vi "Treat DIGITAL variables.vi"(0 "Analog Variable info fixed":T3[](array[typedef]), 1 "Common alarm handling(F)":bool, 5 "All issues in Alm list":bool, 7 "Status Values":T13[](array[typedef]), 9 "Variabel start index":i32, 11 "error In":errorcluster, 12 "Analog Variable info Settings":T6[](array[typedef])) -> (3 "Categorized  Status":T1[](array[typedef]), 4 "Digital Variable Display":T10[](array[typedef]), 6 "Action":T8, 8 "Digital status Values":T13[](array[typedef]), 10 "Alarms":bool[](array[boolean]), 14 "Issue Alarm strings":string[][](array[string]), 15 "error out":errorcluster)   [LabVIEW 2011]
uses:
  Action List.ctl
  Status Digitalish.ctl
  Digital GUI/Digital Display cluster.ctl
  Digital GUI/Digital Disp small indicator.ctl
  GUI/Status indicator white.ctl
  User Setting DigitalChannel.ctl
  Alarm Responce.ctl
  Alarm Responce dig.ctl
  Fixed Digital Channel Definition.ctl
  Update frequensies.ctl
  Channel catagory Enum.ctl
  Catagorised alarm state.ctl
  GUI/Status Indikator Helper.ctl
  Application Structure/Options/Action GFV Settings.ctl
  emi cndiates/E&S/reate/S&E Digital Alarm Type.ctl
  emi Lib/System 01/0 - General/emi_Read System ID.vi
  <vilib>/Utility/VariantDataType/GetNumericInfo.vi
  emi Lib/System 01/0 - General/Private/_emi_GFV System ID.vi
  emi Lib/System 01/0 - General/S&E reporting/Private/_emi_S&E Q Generator.vi
  <vilib>/Utility/error.llb/Clear Errors.vi
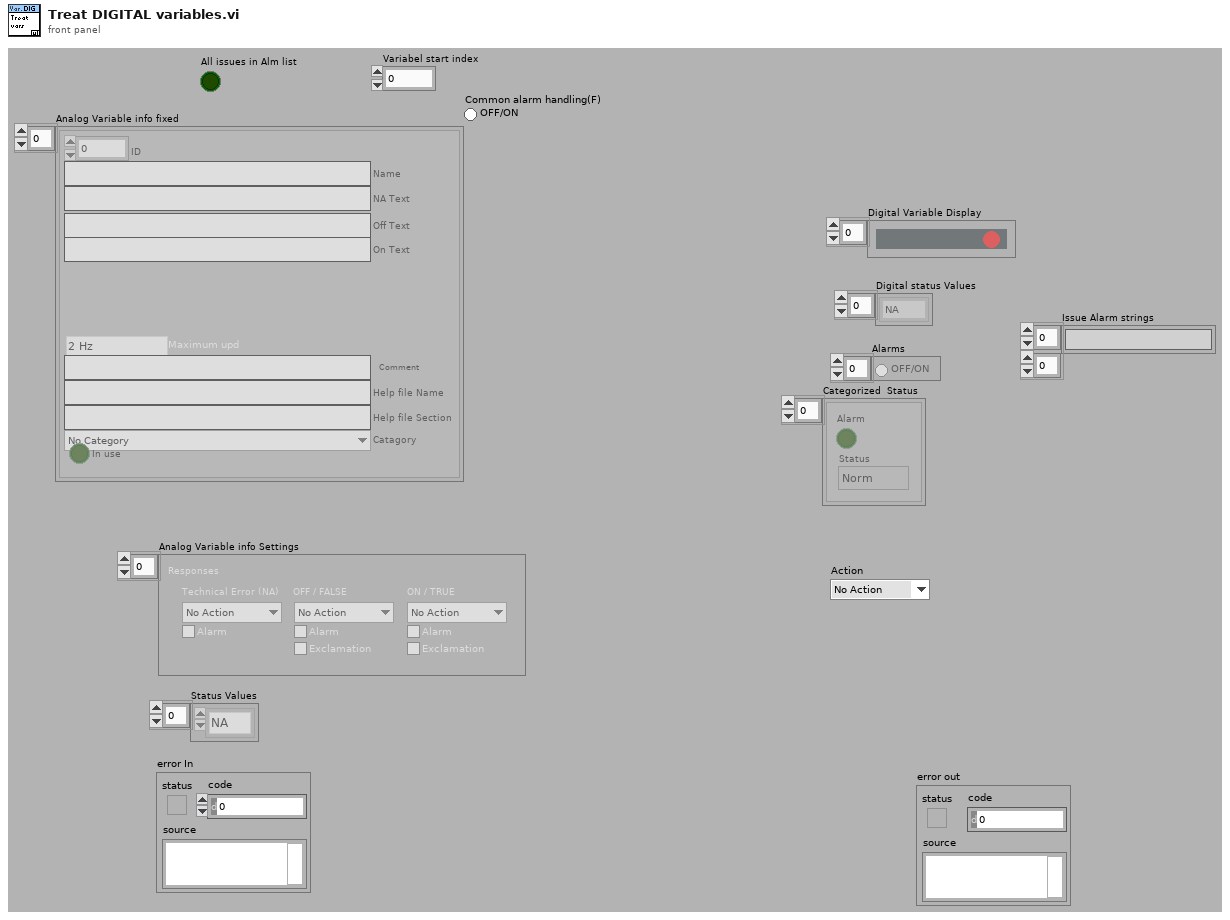
[diagram p1: front panel]
types:
  T1 = typedef "Catagorised alarm state.ctl" = cluster{"Alarm":bool, "Status":T2}
  T2 = typedef "Status Indikator Helper.ctl" = enum16{"Norm", "L", "H", "LL", "HH", "Value", "Technical"}
  T3 = typedef "Fixed Digital Channel Definition.ctl" = cluster{"ID":u16, "Name":string, "NA Text":string, "Off Text":string, "On Text":string, "Maximum upd":T4, "Comment":string, "Help file Name":string, "Help file Section ":string, "Catagory":T5, "In use":bool}
  T4 = typedef "Update frequensies.ctl" = enum16{"2 Hz", "1 Hz", "0.1 Hz"}
  T5 = typedef "Channel catagory Enum.ctl" = enum16{"No Category", "Power", "Temperature", "Pressure"}
  T6 = typedef "User Setting DigitalChannel.ctl" = cluster{"Responses":cluster{"Technical Error (NA)":T7, "OFF / FALSE":T9, "ON / TRUE":T9}}
  T7 = typedef "Alarm Responce.ctl" = cluster{"Action":T8, "Alarm":bool}
  T8 = typedef "Action List.ctl" = enum16{"No Action", "Stop Motor", "Turn Off HV"}
  T9 = typedef "Alarm Responce dig.ctl" = cluster{"Action":T8, "Alarm":bool, "Exclamation":bool}
  T10 = typedef "Digital Display cluster.ctl" = cluster{"ON/OFF TEXT":string, "Val":T11, "Status":T12}
  T11 = typedef "Digital Disp small indicator.ctl" = u16
  T12 = typedef "Status indicator white.ctl" = u16
  T13 = typedef "Status Digitalish.ctl" = enum16{"NA", "False", "True"}
  T14 = typedef "Action GFV Settings.ctl" = enum16{"Init", "Get From INI", "Put In INI", "Get Settings", "Get Update Index", "Set Setting"}
  T15 = typedef "Options  All pages and custom.ctl" = cluster{"P 1 (App)":T16, "P 2":T17, "P 3":T18, "P 4":T21, "P 5":T26, "P 6 (Err)":T27, "P 7 (Expert)":T28, "P 8 (Depth)":T30, "C 1":T31, "C 2":T32}
  T16 = typedef "Options Page 1 (App).ctl" = cluster{"Result files":path, "PCP Interface":string, "Tractor/Stroker Interface":string, "Tractor Interface":string, "Modem Status Interface":string, "Audible Alarm":bool, "Force alarm on Technical":bool, "Force alarm on HH":bool, "Force alarm on LL":bool, "Force alarm on H":bool, "Force alarm on L":bool}
  T17 = typedef "Options Page 2.ctl" = cluster{"Solenoid & Relay latching time":u16, "Tractor relay 1":dbl, "Tractor relay 2":dbl, "Tractor Solenoid limit":dbl}
  T18 = typedef "Options Page 3.ctl" = cluster{"Min resistance":dbl, "Max resistance":dbl, "Head voltage range":T19, "Max voltage jump":dbl, "Maximum resistance change":dbl, "Start Telemetry Voltage":dbl, "Start Telemetry Timeout":dbl, "Start Motor Voltage":dbl, "Stop Motor Voltage":dbl, "Pass Mode Warning Voltage":dbl, "Relay Switch Voltage":dbl, "Relay Status Loss Voltage":dbl, "Samples to average":i32, "PSU type DO NOT USE":T20, "Magna OVP":dbl, "Magna Current Limit":dbl}
  T19 = typedef "PCP type List.ctl" = enum16{"0 - 350V", "0 - 450V", "0 - 600V"}
  T20 = typedef "PSU Type.ctl" = enum16{"Unipower", "Magna 8.3A", "Magna 12A", "None"}
  T21 = typedef "Options Page 4.ctl" = cluster{"Solenoid & Relay latching time":u16, "Stroker relay 1":dbl, "Stroker Relay 2":dbl, "Stroker Solenoid limit":dbl, "Force det.":T22, "Stroke force lim.":dbl, "Anchor Enabled Pressure":dbl, "Tacometer puls":dbl, "Default anchor behavior":T23, "Default stroker behavior":T24, "Default stroker force limit (tonne)":dbl, "Slips Size":T25}
  T22 = typedef "Stroke force selector.ctl" = enum16{"Stroke in = node 1", "Strok out = node 1"}
  T23 = typedef "Default anchor behavior.ctl" = enum16{"Do nothing", "Set Anchor", "Release Anchor"}
  T24 = typedef "Default stroker behavior.ctl" = enum16{"Do nothing", "Stop", "Go Out", "Go In"}
  T25 = typedef "Slips Type Radio.ctl" = enum32{"No Selection", "338 MRS", "3,9 MRS"}
  T26 = typedef "Options Page 5.ctl" = cluster{"Solenoid & Relay latching time":u16, "Driller relay 1":dbl, "Driller Relay 2":dbl, "Driller  Solenoid limit":dbl}
  T27 = typedef "Options Page 6 (Err).ctl" = cluster{"Error and event files":path}
  T28 = typedef "Options Page 7 (Expert).ctl" = cluster{"Show Debug":bool, "Log debug messages":bool, "Additional debug messages":bool, "Start Beagle with Simulator data":bool, "Workshop mode":bool, "Modem baud":u16, "enumCANCOM":bool, "Modem sim":T29, "Telemetry Timeout Disable":i32, "Buffer size":i32, "Upd regular data":bool, "Cable comp":cluster{"VMOD1 Voltage(V)":dbl, "VMOD2 Voltage(V)":dbl}}
  T29 = typedef "Modem simulation setup.ctl" = cluster{"Modem dealay sim":bool, "Sim baud Tx":u16, "Bit Error fraction Tx":dbl, "Sim baud Rx":u16, "Bit Error fraction Rx":dbl}
  T30 = typedef "Options Page 8 (Depth).ctl" = cluster{"Winch Spool Circumference":dbl, "Winch Pulses per Revolution":dbl, "Current Depth":dbl}
  T31 = typedef "Options Custom 1.ctl" = cluster{"Depth Updated":bool, "Depth Offset":dbl}
  T32 = typedef "Options Custom 2.ctl" = cluster{"Placeholder":bool}
  T33 = typedef "S&E Digital Alarm Type.ctl" = cluster{"Alarm":bool, "Enum":T2, "Value":T13, "Source name":string, "Status text":string}
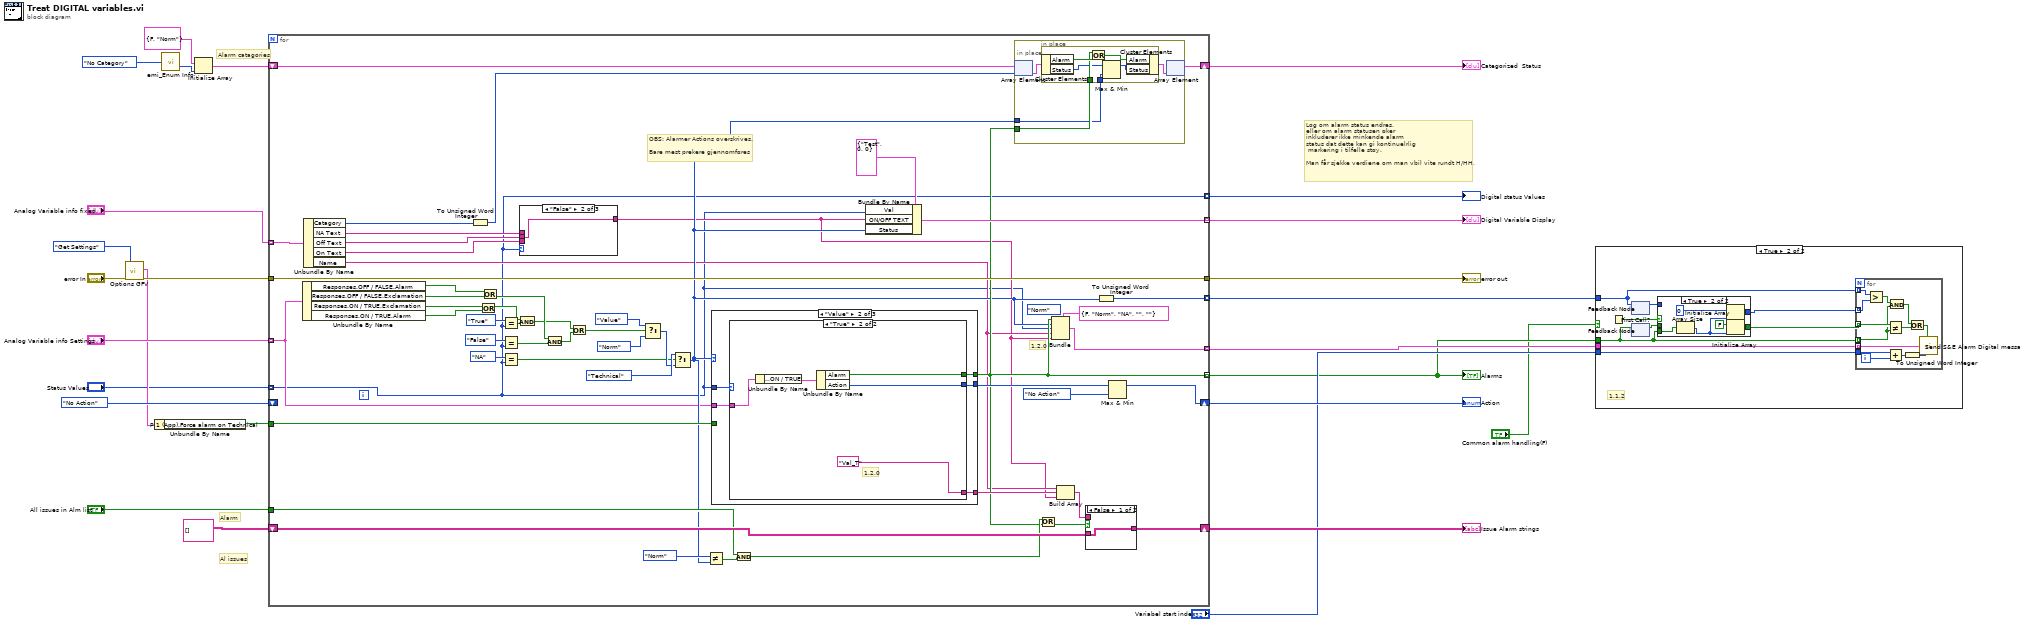
[diagram p0: block diagram]
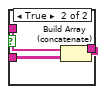
[diagram p6: hidden frame]
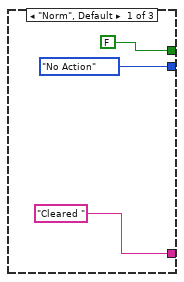
[diagram p7: hidden frame]
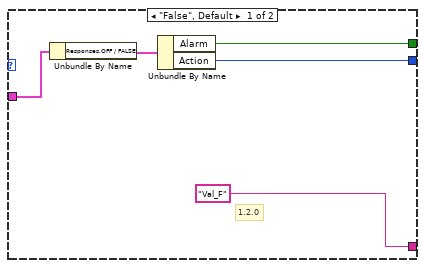
[diagram p8: hidden frame]
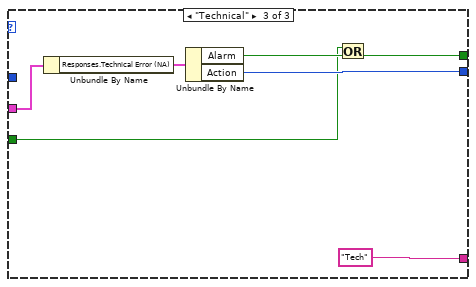
[diagram p9: hidden frame]
diagram:
  # "Log om alarm status endres, \neller om alarm statusen øker\ninkluderer ikke minkende alarm \nstatus dat dette kan gi kontinuelrlig\n markering i tilfelle støy.\n\nMan får sjekke verdiene om man vbil vite rundt H/HH,"
  # "Al issues"
  # "Alarm"
  # "Alarm catagories"
  n1 = call "Options GFV.vi"("error in (no error)"="error In", "Action(Get Settings)"=Action_GFV_Settings."Get Settings") -> ("Options"=w16:T15, "error out"=w18:errorcluster)  [unwired: 15 in, 1 out]
  n2 = Unbundle By Name(w16) -> ("P 1 (App).Force alarm on Technical"=w15:bool)
  n3 = call "emi_Enum Info.vi"("Enum"=Channel_catagory_Enum."No Category" ("Catagory")) -> ("Numb Elements"=w8:i32)  [unwired: 11 in, 3 out]
  n4 = Initialize Array(T1 {"Alarm"=FALSE, "Status"=enum."Norm"} ("catagori"), w8) -> (w6:T1[])
  n5 = for {
    tunnel: "Analog Variable info Settings" -> [w50] mode=indexing
    tunnel: "Analog Variable info fixed" -> [w78] mode=indexing
    tunnel: w18 -> [w74]
    tunnel: [w59] -> w3 mode=indexing
    tunnel: [w75] -> w23 mode=indexing
    tunnel: [w74] -> w24
    shift-right: [w71] -> w26
    shift-left: Action_List."No Action" ("Action") -> [_]
    tunnel: w15 -> [w70]
    shift-right: [w68] -> w14
    shift-left: string[][] [] -> [w67]
    tunnel: "All issues in Alm list" -> [w62]
    tunnel: [w58] -> w11 mode=indexing
    tunnel: [w56] -> w9 mode=indexing
    shift-right: [w54] -> w5
    shift-left: w6 -> [w55]
    tunnel: [w27] -> w4 mode=indexing
    tunnel: "Status Values" -> [w27] mode=indexing
    (unwired) Status_Indikator_Helper."Norm" ("s? t:f")
    # "1.2.0"
    # "OBS: Alarmer Actions overskrives.\n\nBare mest prekere gjennomføres"
    n6 = Unbundle By Name(w50) -> ("Responses.OFF / FALSE.Alarm"=w40:bool, "Responses.OFF / FALSE.Exclamation"=w45:bool, "Responses.ON / TRUE.Exclamation"=w42:bool, "Responses.ON / TRUE.Alarm"=w38:bool)
    n7 = Unbundle By Name(w78) -> ("Catagory"=w33:T5, "NA Text"=w32:string, "Off Text"=w31:string, "On Text"=w30:string, "Name"=w29:string)
    n8 = To Unsigned Word Integer(number=w33) -> (unsigned 16bit integer=w53:u16)
    n9 = Or(x=w42, y=w38) -> (x .or. y?=w39:bool)
    n10 = Or(x=w40, y=w45) -> (x .or. y?=w41:bool)
    n11 = Equal?(x=Status_Digitalish."True", y=w27) -> (x = y?=w43:bool)
    n12 = Equal?(x=Status_Digitalish."False", y=w27) -> (x = y?=w46:bool)
    n13 = Equal?(x=Status_Digitalish."NA", y=w27) -> (x = y?=w48:bool)
    n14 = And(x=w39, y=w43) -> (x .and. y?=w36:bool)
    n15 = case shown="\"False\"" w27 {
      tunnel: w32 -> [w79 _ _]
      tunnel: w31 -> [_ w80 _]
      tunnel: w30 -> [_ _ w81]
      tunnel: [w79 w80 w81] -> w28
      frame "NA", Default {
      }
      frame "False" {
      }
      frame "True" {
      }
    }
    n16 = And(x=w41, y=w46) -> (x .and. y?=w37:bool)
    n17 = Or(x=w36, y=w37) -> (x .or. y?=w35:bool)
    n18 = Select(t=Status_Indikator_Helper."Value" ("Enum"), s=w35, f=Status_Indikator_Helper."Norm" ("Enum")) -> (s? t:f=w52:T2)
    n19 = Select(t=Status_Indikator_Helper."Technical" ("Enum"), s=w48, f=w52) -> (s? t:f=w57:T2)
    n20 = Not Equal?(x=Status_Indikator_Helper."Norm", y=w57) -> (x != y?=w63:bool)
    n21 = case shown="\"Value\"" w57 {
      tunnel: w50 -> [_ w103 w120]
      tunnel: [Action_List."No Action" ("LL.Action") w101 w117] -> w73
      tunnel: [FALSE w102 w116] -> w59
      tunnel: w70 -> [_ _ w115]
      tunnel: ["Cleared " w100 "Tech"] -> w69
      tunnel: w27 -> [_ w99 _]
      frame "Norm", Default {
      }
      frame "Value" {
        n22 = case shown="\"True\"" w99 {
          tunnel: w103 -> [w108 w113]
          tunnel: [w106 w111] -> w102
          tunnel: [w105 w110] -> w101
          tunnel: ["Val_F" "Val_T"] -> w100
          frame "False", Default {
            # "1.2.0"
            n23 = Unbundle By Name(w108) -> ("Responses.OFF / FALSE"=w107:T9)
            n24 = Unbundle By Name(w107) -> ("Alarm"=w106:bool, "Action"=w105:T8)
          }
          frame "True" {
            # "1.2.0"
            n25 = Unbundle By Name(w113) -> ("Responses.ON / TRUE"=w112:T9)
            n26 = Unbundle By Name(w112) -> ("Alarm"=w111:bool, "Action"=w110:T8)
          }
        }
      }
      frame "Technical" {
        n27 = Unbundle By Name(w120) -> ("Responses.Technical Error (NA)"=w119:T7)
        n28 = Unbundle By Name(w119) -> ("Alarm"=w118:bool, "Action"=w117:T8)
        n29 = Or(x=w115, y=w118) -> (x .or. y?=w116:bool)
      }
    }
    n30 = And(x=w62, y=w63) -> (x .and. y?=w61:bool)
    n31 = Bundle By Name(cluster=T10 {"ON/OFF TEXT"="Test", "Val"=0, "Status"=0} ("Depth"), "Val"=w27, "ON/OFF TEXT"=w28, "Status"=w57) -> (w75:T10)
    n32 = in-place {
      in-place-border: w57 -> [w86]
      in-place-border: w59 -> [w87]
      n33 = in-place-array #1(w55, w53) -> (w89:T1)
      n34 = in-place {
        in-place-border: w87 -> [w93]
        in-place-border: w86 -> [w91]
        n35 = in-place-cluster #2(w89) -> ("Alarm"=w95:bool, "Status"=w92:T2)
        n36 = Or(x=w93, y=w95) -> (x .or. y?=w94:bool)
        n37 = Max & Min(x=w92, y=w91) -> (max(x,y)=w90:u16)  [unwired: 1 out]
        n38 = in-place-cluster #2("Alarm"=w94, "Status"=w90) -> (w88:T1)
      }
      n39 = in-place-array #1(w88) -> (w54:T1[])  [unwired: 1 out]
    }
    n40 = Or(x=w61, y=w59) -> (x .or. y?=w65:bool)
    n41 = Bundle(cluster=T33 {"Alarm"=FALSE, "Enum"=enum."Norm", "Value"=enum."NA", "Source name"="", "Status text"=""} ("S&E Alarm"), "Alarm"=w59, "Enum"=w57, "Value"=w27, "Source name"=w29, "Status text"=w28) -> (w58:T33)
    n42 = Build Array(w29, w69, w28) -> (w66:string[])
    n43 = case shown="False" w65 {
      tunnel: [w82 w85] -> w68
      tunnel: w67 -> [w82 w84]
      tunnel: w66 -> [_ w83]
      frame False {
      }
      frame True {
        n44 = Build Array (concatenate)(w83, w84) -> (w85:string[][])
      }
    }
    n45 = To Unsigned Word Integer(number=w57) -> (unsigned 16bit integer=w56:u16)
    n46 = Max & Min(x=w73, y=Action_List."No Action" ("Action")) -> (max(x,y)=w71:u16)  [unwired: 1 out]
  }
  "Action" <- w26
  "Digital status Values" <- w4
  "error out" <- w24
  "Alarms" <- w3
  "Digital Variable Display" <- w23
  "Issue Alarm strings" <- w14
  "Categorized  Status" <- w5
  n47 = case shown="True" "Common alarm handling(F)" {
    tunnel: w11 -> [_ w129]
    tunnel: "Variabel start index" -> [_ w128]
    tunnel: w9 -> [_ w127]
    tunnel: w3 -> [_ w121]
    frame False {
    }
    frame True {
      # "1.1.2"
      n48 = First Call?() -> (First Call?: T/F=w122:bool)
      n49 = feedback #3() -> (w126:u16[])  [unwired: 1 in]
      n50 = feedback-in #3(w127) -> ()
      n51 = feedback #4() -> (w125:bool[])  [unwired: 1 in]
      n52 = feedback-in #4(w121) -> ()
      n53 = case shown="True" w122 {
        tunnel: w126 -> [w144 _]
        tunnel: w125 -> [w143 _]
        tunnel: [w143 w148] -> w124
        tunnel: [w144 w147] -> w123
        tunnel: w121 -> [_ w145]
        frame False {
        }
        frame True {
          n54 = Array Size(array=w145) -> (size(s)=w150:i32)
          n55 = Initialize Array(u16 0 ("unsigned 16bit integer"), w150) -> (w147:u16[])
          n56 = Initialize Array(FALSE, w150) -> (w148:bool[])
        }
      }
      n57 = for {
        tunnel: w124 -> [w142] mode=indexing
        tunnel: w121 -> [w132] mode=indexing
        tunnel: w129 -> [w136] mode=indexing
        tunnel: w128 -> [w139]
        tunnel: w127 -> [w135] mode=indexing
        tunnel: w123 -> [w134] mode=indexing
        i -> [w140]
        n58 = Greater?(x=w135, y=w134) -> (0:w133:bool)
        n59 = Not Equal?(x=w142, y=w132) -> (x != y?=w141:bool)
        n60 = Add(x=w139, y=w140) -> (x+y=w138:i32)
        n61 = And(x=w133, y=w132) -> (x .and. y?=w131:bool)
        n62 = To Unsigned Word Integer(number=w138) -> (unsigned 16bit integer=w137:u16)
        n63 = Or(x=w131, y=w141) -> (x .or. y?=w130:bool)
        n64 = call "Send S&E Alarm Digital message.vi"("Send(T)"=w130, "S&E Alarm"=w136, "Loc Sub ID"=w137) -> ()  [unwired: 11 in, 2 out]
      }
    }
  }
